vi "Write Samples.vi"(8 "error in (no error)":errorcluster, 10 "Samples":refnum<class "Sample.lvclass">[](array[class]), 11 "Metric Session in":refnum<class "Metric Session.lvclass">) -> (0 "error out":errorcluster, 3 "Metric Session out":refnum<class "Metric Session.lvclass">)   [LabVIEW 2020, in "Metrics.lvlib" / "Metric Session.lvclass"]
uses:
  Metric Session.lvclass
  sample/Sample.lvclass
  Metric Session.lvclass/Metric Session.ctl
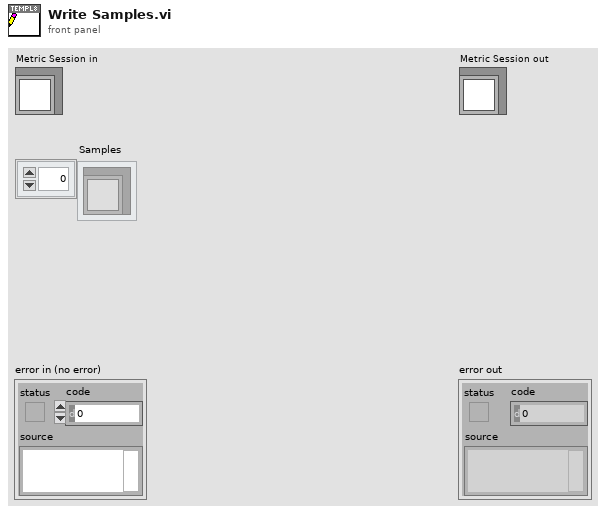
[diagram p1: front panel]
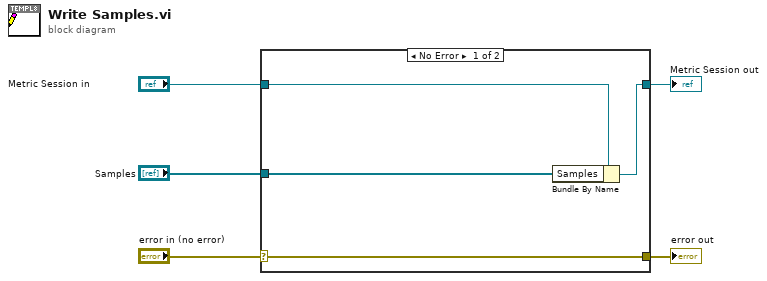
[diagram p0: block diagram]
diagram:
  n1 = case shown="No Error" "error in (no error)" {
    selector: "error in (no error)" -> [w9 w10]
    tunnel: [w9 w10] -> w4
    tunnel: [w7 w11] -> w2
    tunnel: "Metric Session in" -> [w8 w11]
    tunnel: "Samples" -> [w6 _]
    frame No Error {
      n2 = Bundle By Name(cluster=w8, "Samples"=w6) -> (w7:refnum<class "Metric Session.lvclass">)
    }
    frame Error {
    }
  }
  "error out" <- w4
  "Metric Session out" <- w2
